vi "Backup client and server.vi"(8 "error in":errorcluster, 11 "proto File Path":path) -> (0 "error out":errorcluster, 2 "Generated Library Name":string)   [LabVIEW 2021, in "TemplateCoreUtilities.lvlib"]
uses:
  TemplateCoreUtilities.lvlib
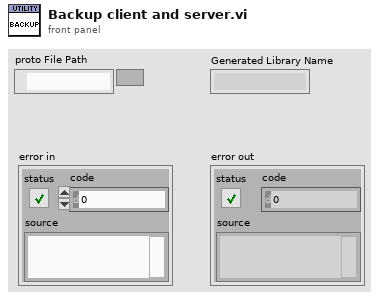
[diagram p1: front panel]
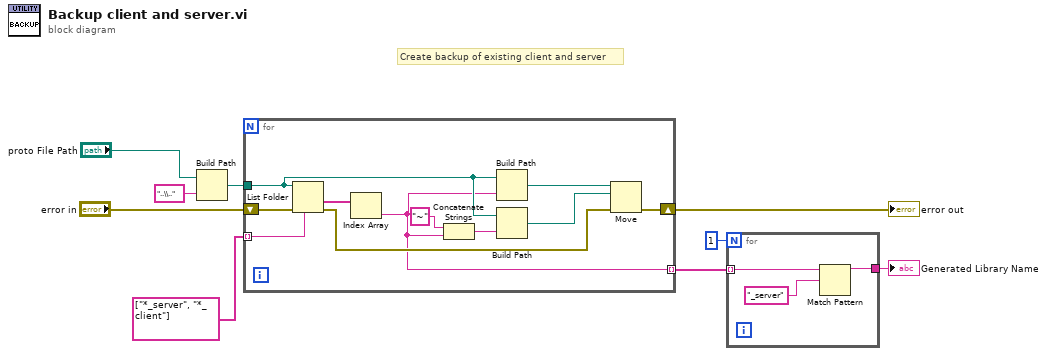
[diagram p0: block diagram]
diagram:
  # "Create backup of existing client and server"
  n1 = Build Path(base path="proto File Path", name or relative path="..\\.." ("String")) -> (appended path=w8:path)
  n2 = for {
    tunnel: w8 -> [w18]
    tunnel: string[] ["*_server", "*_client"] -> [w13] mode=indexing
    shift-right: [w11] -> w3
    shift-left: "error in" -> [w12]
    tunnel: [w10] -> w7 mode=indexing
    n3 = List Folder(path=w18, pattern=w13, error in=w12) -> (folder names=w20:string[], error out=w14:errorcluster)  [unwired: 1 in, 2 out]
    n4 = Index Array(array=w20) -> (element=w10:string)  [unwired: 1 in]
    n5 = Concatenate Strings("~" ("pattern"), w10) -> (w16:string)
    n6 = Build Path(base path=w18, name or relative path=w10) -> (appended path=w19:path)
    n7 = Build Path(base path=w18, name or relative path=w16) -> (appended path=w15:path)
    n8 = Move(source path=w19, error in=w14, 10:w15) -> (error out=w11:errorcluster)  [unwired: 2 in, 2 out]
  }
  "error out" <- w3
  n9 = for {
    N: 1 -> [_]
    tunnel: w7 -> [w23] mode=indexing
    tunnel: [w22] -> w4
    n10 = Match Pattern(string=w23, regular expression="_server" ("pattern")) -> (before substring=w22:string)  [unwired: 1 in, 3 out]
  }
  "Generated Library Name" <- w4
